vi "格式化字符串.vi"(11 "字符串":string) -> (3 "字符串 2":string)   [LabVIEW 2016, in "流量计集成.lvlib" / "WL1A1明渠流量计.lvlib"]
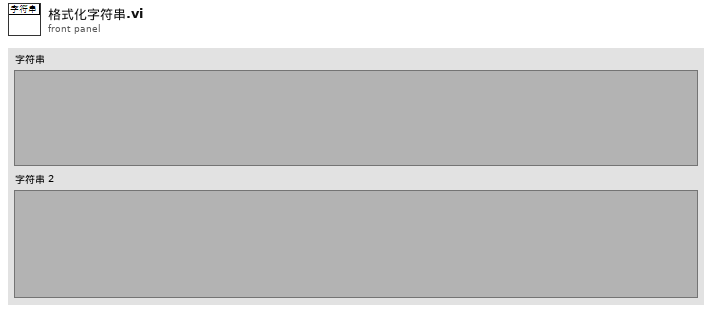
[diagram p1: front panel]
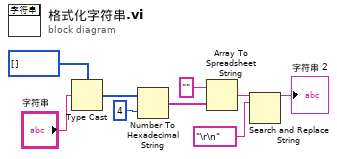
[diagram p0: block diagram]
diagram:
  n1 = Type Cast(type=u16[] [], x="字符串") -> (*(type *) &x=w7:u16[])
  n2 = Number To Hexadecimal String(1:i16 4 ("宽度(-)"), 2:w7) -> (0:w5:string[])
  n3 = Array To Spreadsheet String(array=w5, 3:"" ("格式字符串")) -> (spreadsheet string=w3:string)  [unwired: 1 in]
  n4 = Search and Replace String(input string=w3, search string="\r\n" ("搜索字符串")) -> (result string=→"字符串 2":string)  [unwired: 6 in, 3 out]
